vi "GraphRandG_vs_Parameter.vi"(8 "indices":T1, 9 "AO Amp (V)":dbl[](array[numeric]), 10 "Y vs Parameter":cluster{"X-array":dbl[], "Y-array":dbl[]}[](array[cluster]), 11 "X vs Parameter":cluster{"X-array":dbl[], "Y-array":dbl[]}[](array[cluster])) -> (2 "G(Siemens) vs Parameter":cluster{"X-array":dbl[], dbl[]}[](array[cluster]), 3 "R(Ohms) vs Parameter":cluster{"X-array":dbl[], dbl[]}[](array[cluster]))   [LabVIEW 2019, in "Transport.lvclass"]
uses:
  Transport.lvclass
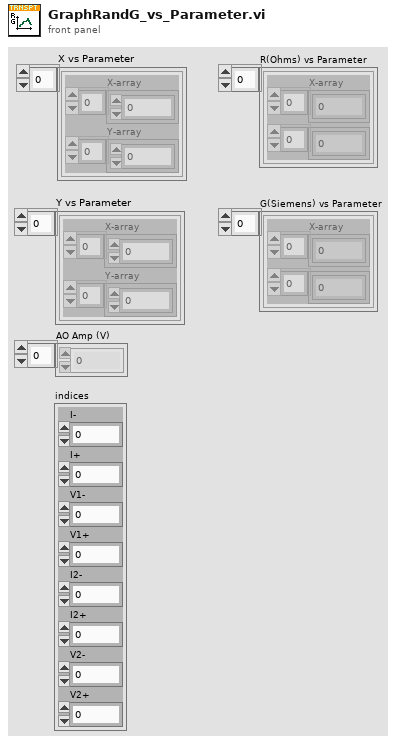
[diagram p1: front panel]
types:
  T1 = cluster{"I-":i32, "I+":i32, "V1-":i32, "V1+":i32, "I2-":i32, "I2+":i32, "V2-":i32, "V2+":i32}
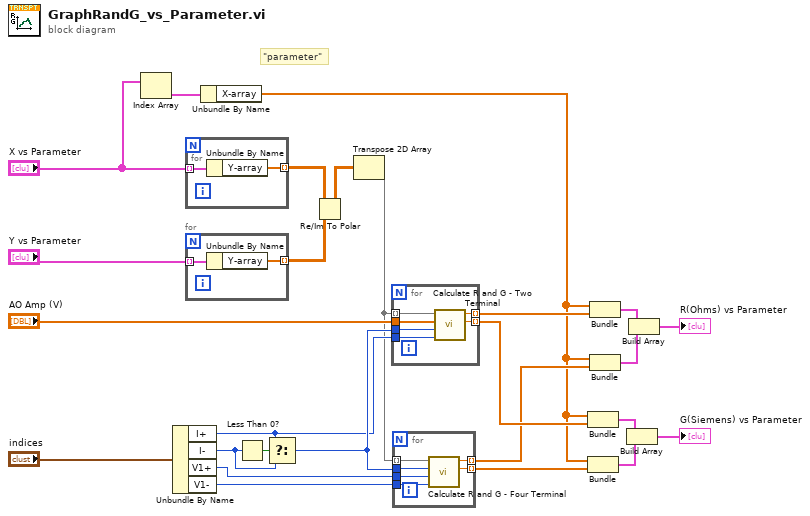
[diagram p0: block diagram]
diagram:
  # "\"parameter\""
  n1 = Index Array(array="X vs Parameter") -> (element=w14:cluster{"X-array":dbl[], "Y-array":dbl[]})  [unwired: 1 in]
  n2 = Unbundle By Name("indices") -> ("I+"=w18:i32, "I-"=w19:i32, "V1+"=w16:i32, "V1-"=w15:i32)
  n3 = for {
    tunnel: "X vs Parameter" -> [w28] mode=indexing
    tunnel: [w27] -> w5 mode=indexing
    n4 = Unbundle By Name(w28) -> ("Y-array"=w27:dbl[])
  }
  n5 = for {
    tunnel: "Y vs Parameter" -> [w30] mode=indexing
    tunnel: [w29] -> w6 mode=indexing
    n6 = Unbundle By Name(w30) -> ("Y-array"=w29:dbl[])
  }
  n7 = Unbundle By Name(w14) -> ("X-array"=w3:dbl[])
  n8 = Less Than 0?(x=w19) -> (x < 0?=w17:bool)
  n9 = Select(t=w18, s=w17, f=w19) -> (s? t:f=w20:i32)
  n10 = Re/Im To Polar(2:w6, 3:w5) -> (1:w4:dbl[][])  [unwired: 1 out]
  n11 = Transpose 2D Array(2D array=w4) -> (transposed array=w1:dbl[][])
  n12 = for {
    tunnel: w18 -> [w36]
    tunnel: w20 -> [w35]
    tunnel: w1 -> [w34] mode=indexing
    tunnel: [w33] -> w22 mode=indexing
    tunnel: [w32] -> w25 mode=indexing
    tunnel: "AO Amp (V)" -> [w31]
    n13 = call "Calculate R and G - Two Terminal.vi"("Vsource"=w36, "Current"=w35, "AO Amp (V)"=w31, "Lockin []"=w34) -> ("G_2T (Siemens)"=w32:dbl, "R_2T (Ohms)"=w33:dbl)  [unwired: 6 in]
  }
  n14 = for {
    tunnel: w15 -> [w42]
    tunnel: w16 -> [w41]
    tunnel: w20 -> [w40]
    tunnel: w1 -> [w39] mode=indexing
    tunnel: [w38] -> w24 mode=indexing
    tunnel: [w37] -> w23 mode=indexing
    n15 = call "Calculate R and G - Four Terminal.vi"("V-"=w42, "V+"=w41, "Current"=w40, "Lockin[ ]"=w39) -> ("G_4T (Siemens)"=w37:dbl, "R_4T (ohms)"=w38:dbl)  [unwired: 4 in, 2 out]
  }
  n16 = Bundle("X-array"=w3, w25) -> (w8:cluster{"X-array":dbl[], dbl[]})  [unwired: 1 in]
  n17 = Bundle("X-array"=w3, w23) -> (w10:cluster{"X-array":dbl[], dbl[]})  [unwired: 1 in]
  n18 = Bundle("X-array"=w3, w22) -> (w12:cluster{"X-array":dbl[], dbl[]})  [unwired: 1 in]
  n19 = Bundle("X-array"=w3, w24) -> (w11:cluster{"X-array":dbl[], dbl[]})  [unwired: 1 in]
  n20 = Build Array(w8, w10) -> (→"G(Siemens) vs Parameter":cluster{"X-array":dbl[], dbl[]}[])
  n21 = Build Array(w12, w11) -> (→"R(Ohms) vs Parameter":cluster{"X-array":dbl[], dbl[]}[])
